vi "room catch or put.vi"(5 "get recy?":bool=TRUE, 7 "first?":bool, 8 "error in (no error)":errorcluster, 9 "Position in":T3, 10 "ff":i32, 11 "main-national data":T1) -> (0 "error out":errorcluster, 1 "Position out":T3, 3 "main-national data out":T1, 4 "finish?":bool)   [LabVIEW 2019]
uses:
  ctl/main data-national.ctl
  ctl/position set.ctl
  subVI/move/position cluster.ctl
  ctl/path name.ctl
  ctl/align type.ctl
  ctl/height.ctl
  ctl/servo act.ctl
panel:
  out "Array":bool[](array[boolean])
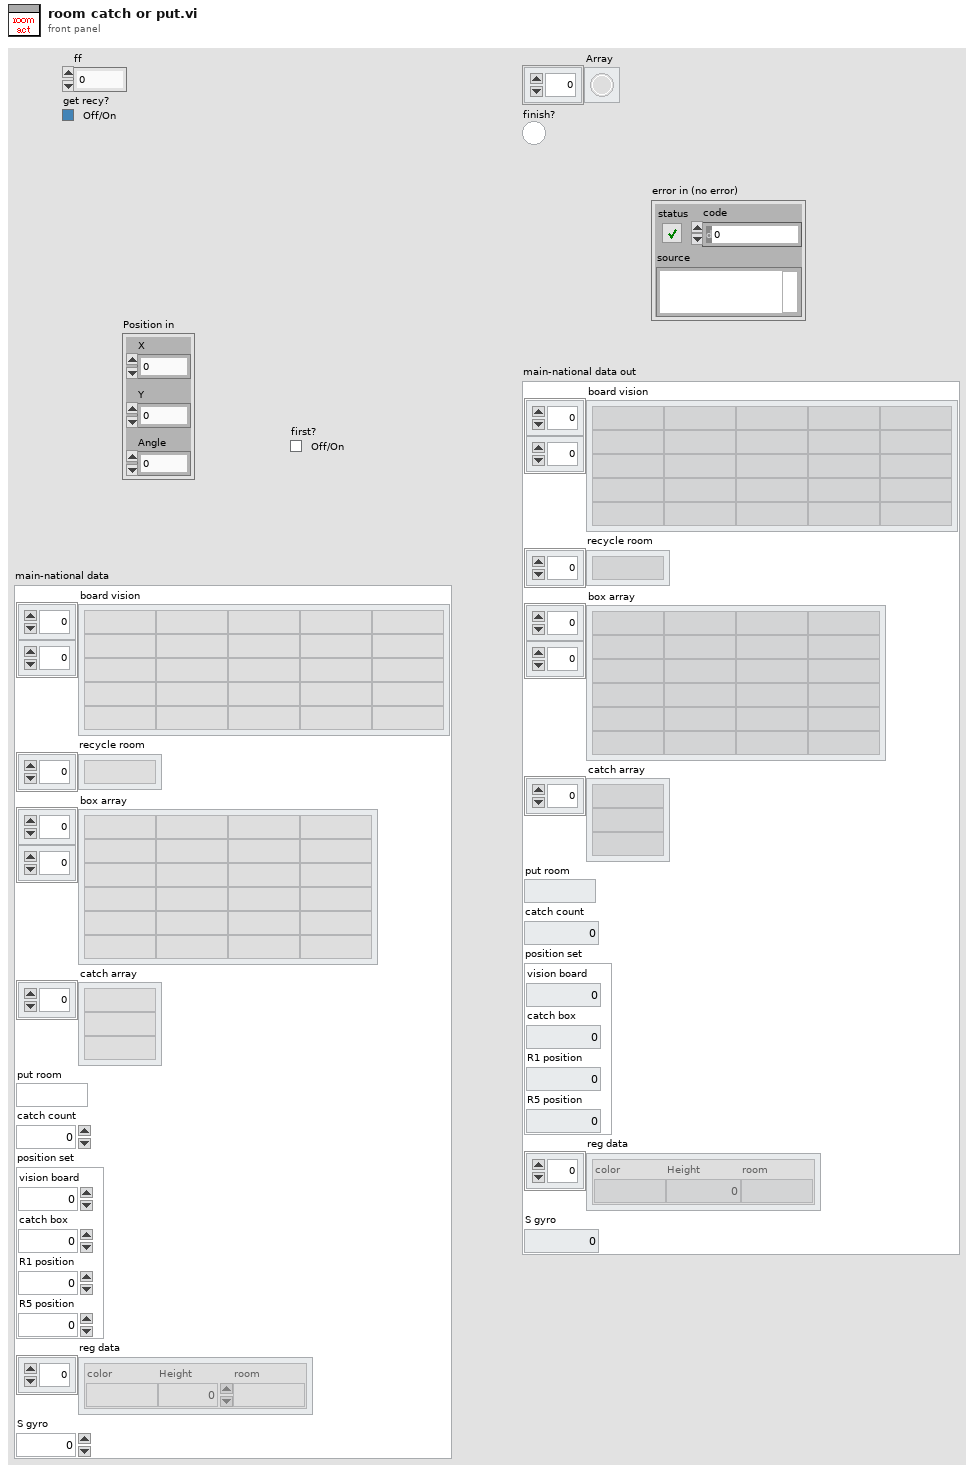
[diagram p1: front panel]
types:
  T1 = typedef "main data-national.ctl" = cluster{"board vision":string[][], "recycle room":string[], "box array":string[][], "catch array":string[], "put room":string, "catch count":dbl, "position set":T2, "reg data":cluster{"color":string, "Height":i32, "room":string}[], "S gyro":dbl}
  T2 = typedef "position set.ctl" = cluster{"vision board":dbl, "catch box":dbl, "R1 position":dbl, "R5 position":dbl}
  T3 = typedef "position cluster.ctl" = cluster{"X":dbl, "Y":dbl, "Angle":dbl}
  T4 = cluster{"color":string, "Height":i32, "room":string}[]
  T5 = typedef "path name.ctl" = enum16{"S - vision board", "vision board - s out", "s out - room center", "room center - R1", "room center - R2", "room center - R3", "room center - R4", "room center - R5", "R1 - room center", "R2 - room center", "R3 - room center", "R4 - room center", "R5 - room center", "room center - S out", "S-out - recycle", "recycle - S-out", "S-out - s", "s - s-out", "board - box", "box - board", "S out - board", "R1 - R1 d", "R5d - R5", "R3.4-R3", "R3 - R3.2", "- align", "- align.5", "R2 - R2.d", "center align"}
  T6 = typedef "align type.ctl" = enum16{"S zone", "box align", "box align contrast", "R1 align", "R5 align", "-> R5 center align", "-> R1 center align"}
  T7 = typedef "servo act.ctl" = enum16{"catch", "relax", "left idle", "center", "red relax", "left reg", "right reg"}
  T8 = typedef "height.ctl" = enum16{"IDLE", "recycle pre-catch", "recycle catch", "recycle zone", "vision height", "box 1", "box 2", "box 3", "box 1 pre", "box 2 pre", "box 3 pre", "reg 1", "reg 2", "reg 1 pre", "reg 2 pre", "put 1", "put 2", "put 3"}
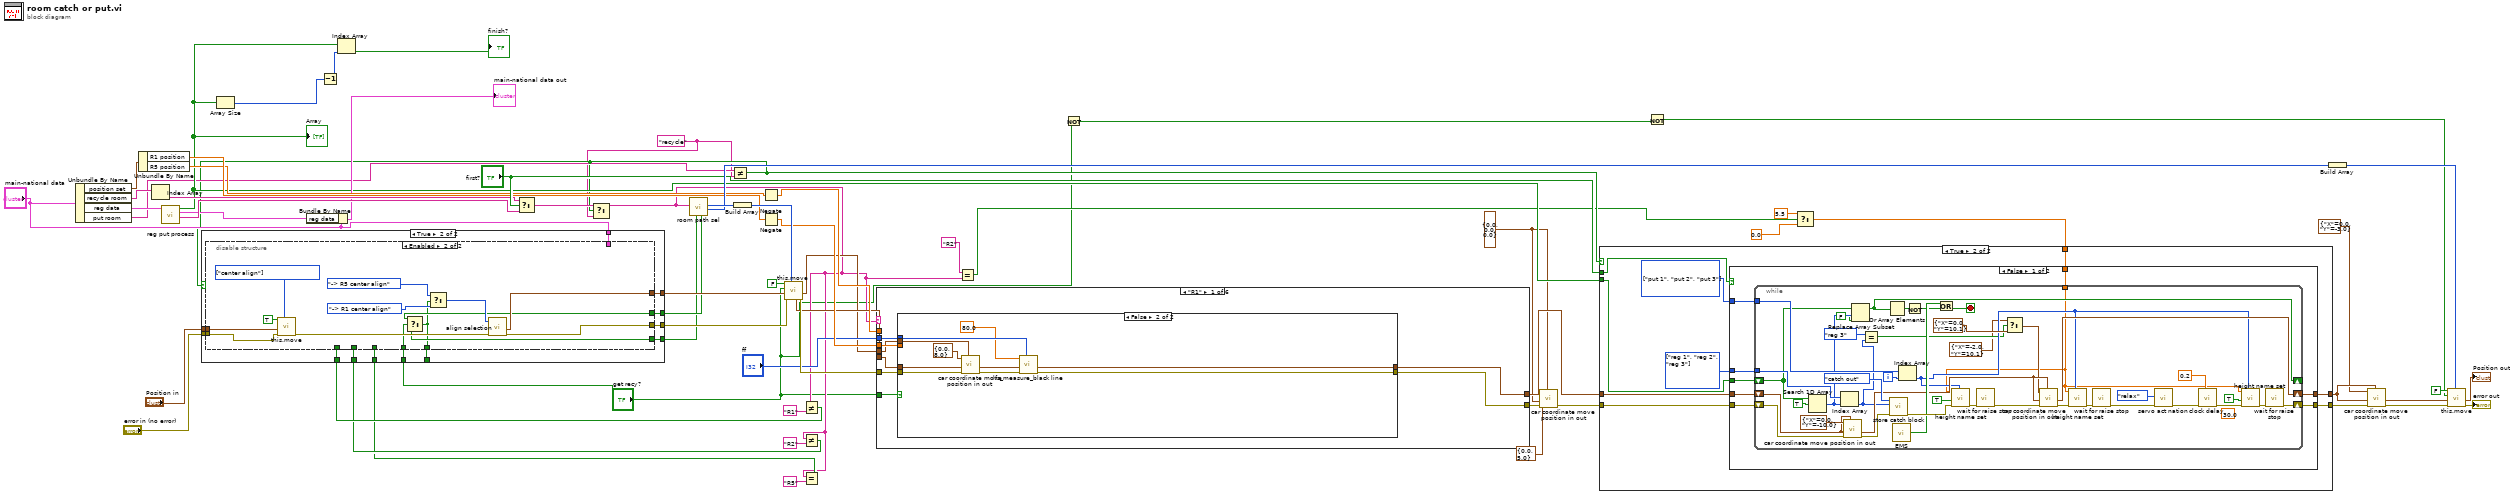
[diagram p0: block diagram]
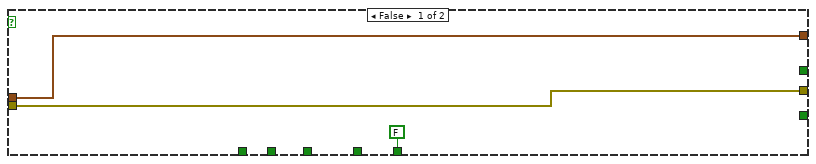
[diagram p2: hidden frame]
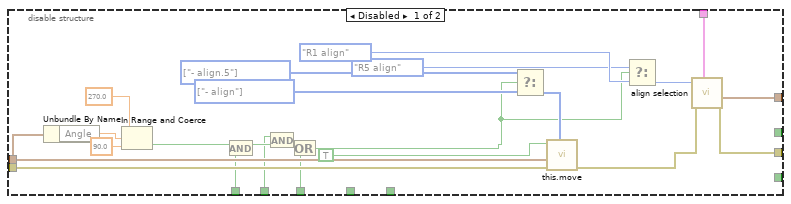
[diagram p3: hidden frame]
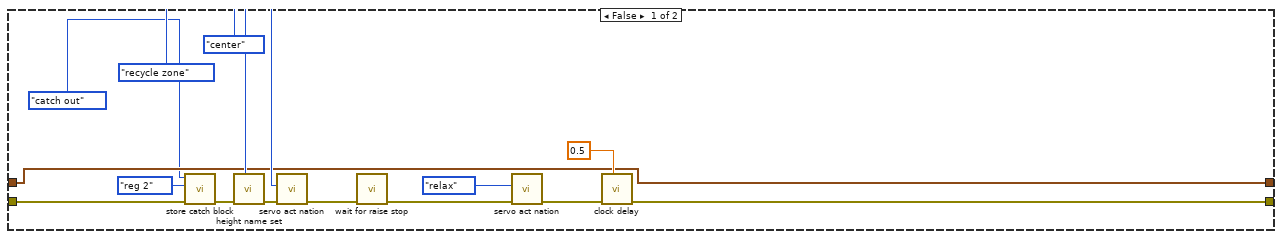
[diagram p4: hidden frame]
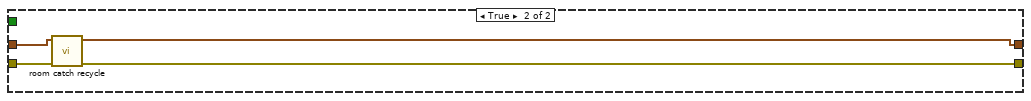
[diagram p5: hidden frame]
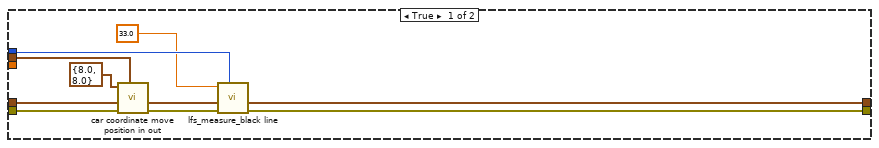
[diagram p6: hidden frame]
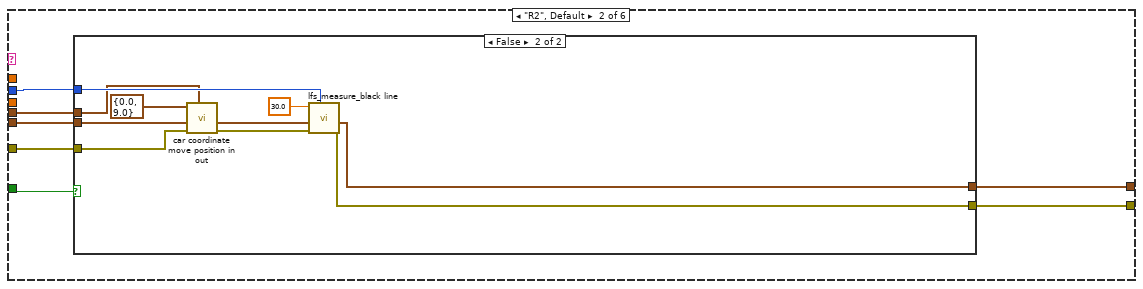
[diagram p7: hidden frame]
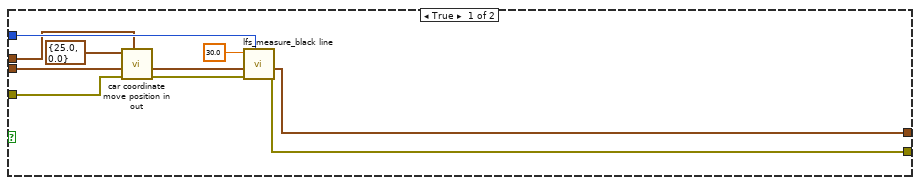
[diagram p8: hidden frame]
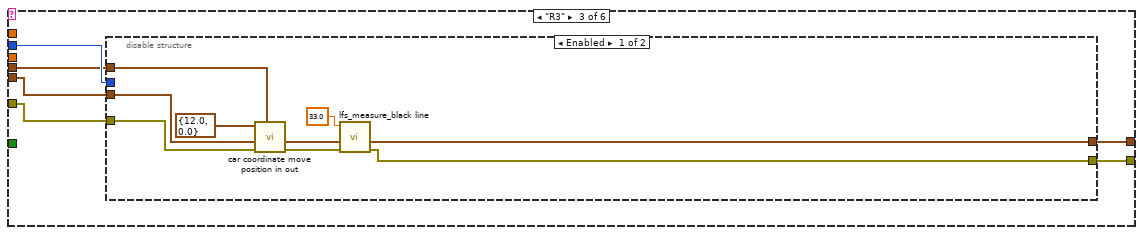
[diagram p9: hidden frame]
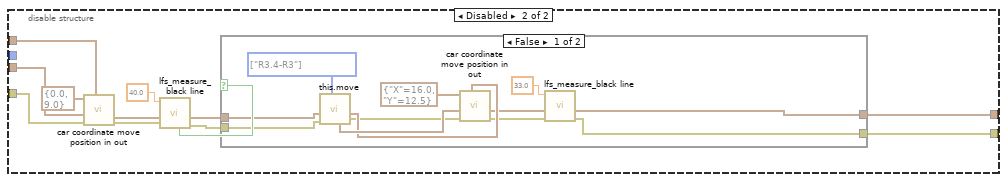
[diagram p10: hidden frame]
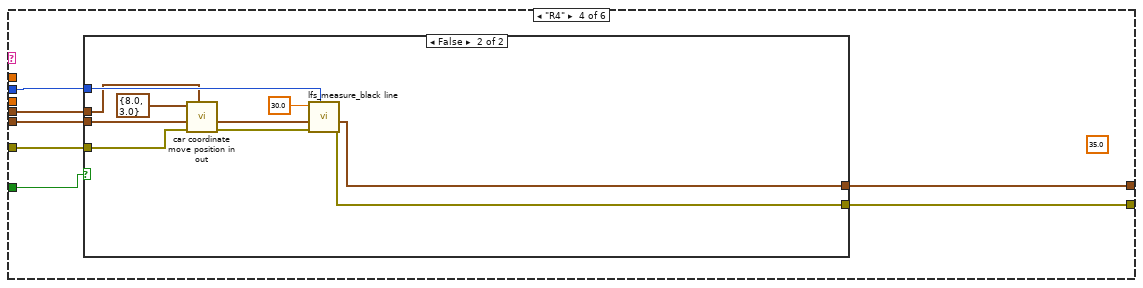
[diagram p12: hidden frame]
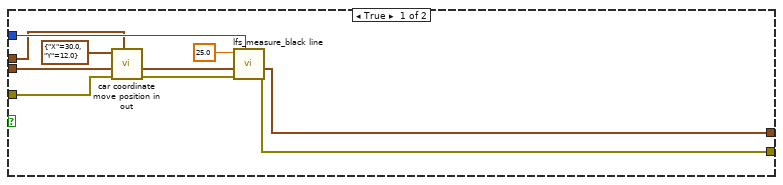
[diagram p13: hidden frame]
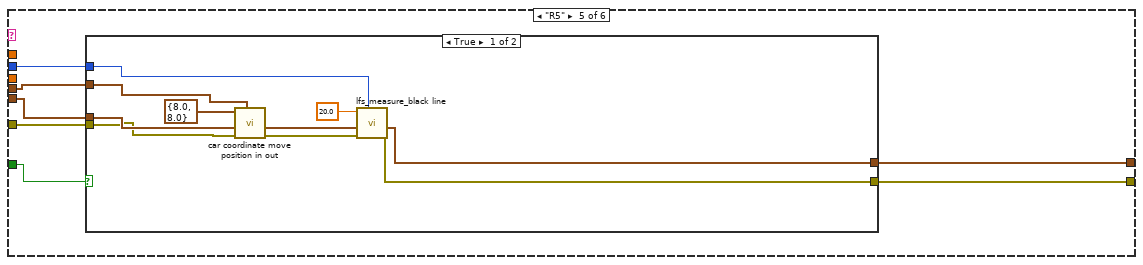
[diagram p14: hidden frame]
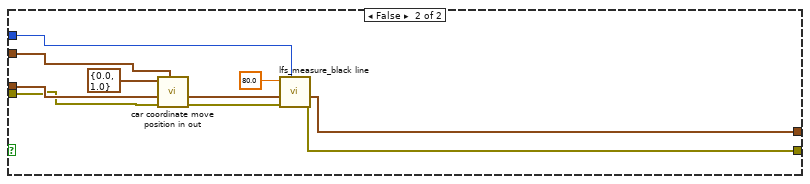
[diagram p15: hidden frame]
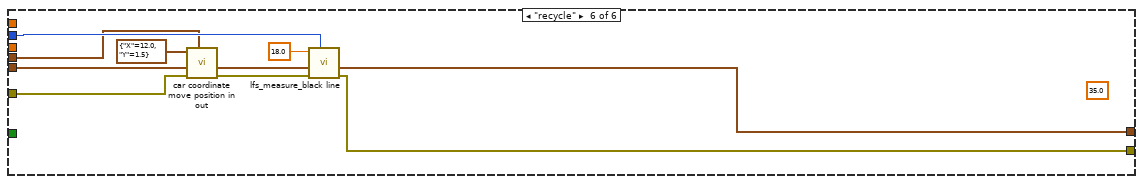
[diagram p16: hidden frame]
diagram:
  w17 = T3 {"X"=0.0, "Y"=0.0, "Angle"=0.0} ("Position in 2")
  w30 = "recycle" ("y")
  n1 = Unbundle By Name("main-national data") -> ("position set"=w52:T2, "recycle room"=w55:string[], "reg data"=w41:T4, "put room"=w32:string)
  n2 = Unbundle By Name(w52) -> ("R1 position"=w51:dbl, "R5 position"=w50:dbl)
  n3 = Index Array(array=w55) -> (element=w47:string)  [unwired: 1 in]
  n4 = call "reg put process.vi"("reg data in"=w41) -> ("room"=w40:string, "reg data out"=w38:T4, "Array"=w34:bool[])  [unwired: 8 in]
  "Array" <- w34
  n5 = Array Size(array=w34) -> (size(s)=w36:i32)
  n6 = Bundle By Name(cluster="main-national data", "reg data"=w38) -> (→"main-national data out":T1)
  n7 = Decrement(x=w36) -> (x-1=w35:i32)
  n8 = Index Array(array=w34, index=w35) -> (element=→"finish?":bool)
  n9 = Select(t=w47, s="first?", f=w40) -> (s? t:f=w53:string)
  n10 = Not Equal?(x=w32, y=w30) -> (x != y?=w31:bool)
  n11 = Select(t=w53, s=w31, f=w30) -> (s? t:f=w10:string)
  n12 = call "room path sel.vi"("room name"=w10) -> ("go next"=w61:T5, "go room path"=w64:T5, "recy dir"=w5:bool, "block dir"=w4:bool)  [unwired: 7 in]
  n13 = Build Array(w64) -> (w63:T5[])
  n14 = Negate(x=w50) -> (-x=w48:dbl)
  n15 = Negate(x=w51) -> (-x=w49:dbl)
  n16 = Not Equal?(x=w10, y="R1") -> (x != y?=w24:bool)
  n17 = Not Equal?(x=w10, y="R2") -> (x != y?=w22:bool)
  n18 = Equal?(x=w10, y="R5") -> (x = y?=w20:bool)
  n19 = case shown="True" w31 {
    tunnel: "Position in" -> [w67 w75]
    tunnel: "error in (no error)" -> [w66 w79]
    tunnel: [w66 w78] -> w43
    tunnel: [w67 w77] -> w42
    tunnel: "main-national data" -> [_ w76]
    tunnel: w24 -> [_ w74]
    tunnel: w22 -> [_ w73]
    tunnel: w20 -> [_ w72]
    tunnel: w5 -> [_ w71]
    tunnel: w4 -> [_ w70]
    tunnel: [FALSE ("block dir") w69] -> _
    tunnel: "get recy?" -> [_ w68]
    frame False {
    }
    frame True {
      n20 = disable-structure shown="Enabled" {
        disable-tunnel: w79 -> [w102 w116]
        disable-tunnel: [w97 w107] -> w78
        disable-tunnel: [w96 w108] -> w77
        disable-tunnel: w76 -> [w95 _]
        disable-tunnel: w75 -> [w92 w115]
        disable-tunnel: w74 -> [w84 _]
        disable-tunnel: w73 -> [w82 _]
        disable-tunnel: w72 -> [w80 _]
        disable-tunnel: w71 -> [_ w106]
        disable-tunnel: w70 -> [_ w105]
        disable-tunnel: [_ w104] -> w69
        disable-tunnel: w68 -> [_ w103]
        frame Disabled {
          w88 = T5[] [enum."- align.5"] items=["S - vision board", "vision board - s out", "s out - room center", "room center - R1", "room center - R2", "room center - R3", "room center - R4", "room center - R5", "R1 - room center", "R2 - room center", "R3 - room center", "R4 - room center", "R5 - room center", "room center - S out", "S-out - recycle", "recycle - S-out", "S-out - s", "s - s-out", "board - box", "box - board", "S out - board", "R1 - R1 d", "R5d - R5", "R3.4-R3", "R3 - R3.2", "- align", "- align.5", "R2 - R2.d", "center align"] ("t")
          w100 = T5[] [enum."- align"] items=["S - vision board", "vision board - s out", "s out - room center", "room center - R1", "room center - R2", "room center - R3", "room center - R4", "room center - R5", "R1 - room center", "R2 - room center", "R3 - room center", "R4 - room center", "R5 - room center", "room center - S out", "S-out - recycle", "recycle - S-out", "S-out - s", "s - s-out", "board - box", "box - board", "S out - board", "R1 - R1 d", "R5d - R5", "R3.4-R3", "R3 - R3.2", "- align", "- align.5", "R2 - R2.d", "center align"] ("path array")
          n21 = Unbundle By Name(w92) -> ("Angle"=w91:dbl)
          n22 = In Range and Coerce(upper limit=270.0, x=w91, lower limit=90.0) -> (In Range?=w87:bool)  [unwired: 1 out]
          n23 = And(x=w87, y=w84) -> (x .and. y?=w85:bool)
          n24 = And(x=w82, y=w85) -> (x .and. y?=w83:bool)
          n25 = Or(x=w83, y=w80) -> (x .or. y?=w81:bool)
          n26 = Select(t=w88, s=w81, f=w100) -> (s? t:f=w93:T5[])
          n27 = call "this.move.vi"("path array"=w93, "error in (no error)"=w102, "Position in"=w92, "enable"=TRUE) -> ("error out"=w98:errorcluster)  [unwired: 4 in, 3 out]
          n28 = Select(t=align_type."R5 align", s=w81, f=align_type."R1 align" ("align type")) -> (s? t:f=w94:T6)
          n29 = call "align selection.vi"("main-national data"=w95, "error in (no error)"=w98, "align type"=w94) -> ("error out"=w97:errorcluster, "Position"=w96:T3)  [unwired: 6 in, 1 out]
        }
        frame Enabled {
          w113 = T5[] [enum."center align"] items=["S - vision board", "vision board - s out", "s out - room center", "room center - R1", "room center - R2", "room center - R3", "room center - R4", "room center - R5", "R1 - room center", "R2 - room center", "R3 - room center", "R4 - room center", "R5 - room center", "room center - S out", "S-out - recycle", "recycle - S-out", "S-out - s", "s - s-out", "board - box", "box - board", "S out - board", "R1 - R1 d", "R5d - R5", "R3.4-R3", "R3 - R3.2", "- align", "- align.5", "R2 - R2.d", "center align"] ("path array")
          n30 = call "this.move.vi"("path array"=w113, "error in (no error)"=w116, "Position in"=w115, "enable"=TRUE) -> ("error out"=w112:errorcluster)  [unwired: 4 in, 3 out]
          n31 = Select(t=w106, s=w103, f=w105) -> (s? t:f=w104:bool)
          n32 = Select(t=align_type."-> R5 center align" ("align type"), s=w104, f=align_type."-> R1 center align" ("align type")) -> (s? t:f=w111:T6)
          n33 = call "align selection.vi"("error in (no error)"=w112, "align type"=w111) -> ("error out"=w107:errorcluster, "Position"=w108:T3)  [unwired: 7 in, 1 out]
        }
      }
    }
  }
  n34 = call "this.move.vi"("path array"=w63, "error in (no error)"=w43, "Position in"=w42, "recy?"="get recy?", "enable"=FALSE) -> ("error out"=w62:errorcluster, "Position out"=w18:T3, "Position out 2"=w19:T3)  [unwired: 3 in, 1 out]
  n35 = case shown="\"R1\"" w10 {
    tunnel: w62 -> [w123 w151 w176 w218 w245 w274]
    tunnel: w19 -> [w124 w150 w177 w219 w246 w275]
    tunnel: [w122 w148 w174 w216 w244 w270] -> w26
    tunnel: [w121 w149 w175 w217 w243 w269] -> w29
    tunnel: w49 -> [w120 _ _ _ _ _]
    tunnel: w48 -> [_ _ _ _ _ _]
    tunnel: "ff" -> [w119 w147 w173 w215 w242 w268]
    tunnel: w18 -> [w118 w146 w172 w214 w241 w267]
    tunnel: "get recy?" -> [w117 w145 _ w213 w240 _]
    frame "R1" {
      n36 = case shown="False" w117 {
        tunnel: w124 -> [w131 w141]
        tunnel: w123 -> [w130 w140]
        tunnel: [w129 w139] -> w122
        tunnel: [w128 w138] -> w121
        tunnel: w120 -> [_ _]
        tunnel: w119 -> [w127 w137]
        tunnel: w118 -> [w126 w136]
        frame True {
          n37 = call "car coordinate move position in out.vi"("Position in 2"=w126, "error in (no error)"=w130, "Position in"=w131, "move"=cluster{"X":dbl, "Y":dbl} {"X"=8.0, "Y"=8.0} ("R1 move")) -> ("error out"=w133:errorcluster, "Position out"=w134:T3)  [unwired: 6 in]
          n38 = call "lfs_measure_black line.vi"("ff"=w127, "error in (no error)"=w133, "Position in"=w134, "limit"=33.0) -> ("error out"=w128:errorcluster, "Position  out"=w129:T3)  [unwired: 3 in, 3 out]
        }
        frame False {
          n39 = call "car coordinate move position in out.vi"("Position in 2"=w136, "error in (no error)"=w140, "Position in"=w141, "move"=cluster{"X":dbl, "Y":dbl} {"X"=0.0, "Y"=8.0} ("R1 move")) -> ("error out"=w143:errorcluster, "Position out"=w144:T3)  [unwired: 6 in]
          n40 = call "lfs_measure_black line.vi"("ff"=w137, "error in (no error)"=w143, "Position in"=w144, "limit"=80.0) -> ("error out"=w138:errorcluster, "Position  out"=w139:T3)  [unwired: 3 in, 3 out]
        }
      }
    }
    frame "R2", Default {
      n41 = case shown="False" w145 {
        tunnel: w151 -> [w161 w171]
        tunnel: w150 -> [w160 w170]
        tunnel: [w159 w169] -> w149
        tunnel: [w158 w168] -> w148
        tunnel: w147 -> [w157 w167]
        tunnel: w146 -> [w156 w166]
        frame True {
          n42 = call "car coordinate move position in out.vi"("Position in 2"=w156, "error in (no error)"=w161, "Position in"=w160, "move"=cluster{"X":dbl, "Y":dbl} {"X"=25.0, "Y"=0.0}) -> ("error out"=w154:errorcluster, "Position out"=w153:T3)  [unwired: 6 in]
          n43 = call "lfs_measure_black line.vi"("ff"=w157, "error in (no error)"=w154, "Position in"=w153, "limit"=30.0) -> ("error out"=w159:errorcluster, "Position  out"=w158:T3)  [unwired: 3 in, 3 out]
        }
        frame False {
          n44 = call "car coordinate move position in out.vi"("Position in 2"=w166, "error in (no error)"=w171, "Position in"=w170, "move"=cluster{"X":dbl, "Y":dbl} {"X"=0.0, "Y"=9.0}) -> ("error out"=w164:errorcluster, "Position out"=w163:T3)  [unwired: 6 in]
          n45 = call "lfs_measure_black line.vi"("ff"=w167, "error in (no error)"=w164, "Position in"=w163, "limit"=30.0) -> ("error out"=w169:errorcluster, "Position  out"=w168:T3)  [unwired: 3 in, 3 out]
        }
      }
    }
    frame "R3" {
      n46 = disable-structure shown="Enabled" {
        disable-tunnel: w177 -> [w182 w197]
        disable-tunnel: w176 -> [w181 w198]
        disable-tunnel: [w180 w188] -> w175
        disable-tunnel: [w179 w187] -> w174
        disable-tunnel: w173 -> [_ _]
        disable-tunnel: w172 -> [w178 w196]
        frame Enabled {
          n47 = call "car coordinate move position in out.vi"("Position in 2"=w178, "error in (no error)"=w181, "Position in"=w182, "move"=cluster{"X":dbl, "Y":dbl} {"X"=12.0, "Y"=0.0}) -> ("error out"=w185:errorcluster, "Position out"=w184:T3)  [unwired: 6 in]
          n48 = call "lfs_measure_black line.vi"("error in (no error)"=w185, "Position in"=w184, "limit"=33.0) -> ("error out"=w180:errorcluster, "Position  out"=w179:T3)  [unwired: 4 in, 3 out]
        }
        frame Disabled {
          n49 = call "car coordinate move position in out.vi"("Position in 2"=w196, "error in (no error)"=w198, "Position in"=w197, "move"=cluster{"X":dbl, "Y":dbl} {"X"=0.0, "Y"=9.0}) -> ("error out"=w192:errorcluster, "Position out"=w193:T3)  [unwired: 6 in]
          n50 = call "lfs_measure_black line.vi"("error in (no error)"=w192, "Position in"=w193, "limit"=40.0) -> ("error out"=w189:errorcluster, "Position  out"=w190:T3, "black?"=w191:bool)  [unwired: 4 in, 2 out]
          n51 = case shown="False" w191 {
            tunnel: w190 -> [w209 w212]
            tunnel: w189 -> [w208 w211]
            tunnel: [w200 w211] -> w188
            tunnel: [w199 w212] -> w187
            frame False {
              w210 = T5[] [enum."R3.4-R3"] items=["S - vision board", "vision board - s out", "s out - room center", "room center - R1", "room center - R2", "room center - R3", "room center - R4", "room center - R5", "R1 - room center", "R2 - room center", "R3 - room center", "R4 - room center", "R5 - room center", "room center - S out", "S-out - recycle", "recycle - S-out", "S-out - s", "s - s-out", "board - box", "box - board", "S out - board", "R1 - R1 d", "R5d - R5", "R3.4-R3", "R3 - R3.2", "- align", "- align.5", "R2 - R2.d", "center align"] ("path array")
              n52 = call "this.move.vi"("path array"=w210, "error in (no error)"=w208, "Position in"=w209) -> ("error out"=w204:errorcluster, "Position out"=w205:T3, "Position out 2"=w206:T3)  [unwired: 5 in, 1 out]
              n53 = call "car coordinate move position in out.vi"("Position in 2"=w205, "error in (no error)"=w204, "Position in"=w206, "move"=cluster{"X":dbl, "Y":dbl} {"X"=16.0, "Y"=12.5}) -> ("error out"=w203:errorcluster, "Position out"=w202:T3)  [unwired: 6 in]
              n54 = call "lfs_measure_black line.vi"("error in (no error)"=w203, "Position in"=w202, "limit"=33.0) -> ("error out"=w200:errorcluster, "Position  out"=w199:T3)  [unwired: 4 in, 3 out]
            }
            frame True {
            }
          }
        }
      }
    }
    frame "R4" {
      (unwired) 35.0 ("speed")
      n55 = case shown="False" w213 {
        tunnel: w219 -> [w225 w235]
        tunnel: w218 -> [w224 w234]
        tunnel: [w223 w233] -> w217
        tunnel: [w222 w232] -> w216
        tunnel: w215 -> [w221 w231]
        tunnel: w214 -> [w220 w230]
        frame True {
          n56 = call "car coordinate move position in out.vi"("Position in 2"=w220, "error in (no error)"=w224, "Position in"=w225, "move"=cluster{"X":dbl, "Y":dbl} {"X"=30.0, "Y"=12.0}) -> ("error out"=w228:errorcluster, "Position out"=w229:T3)  [unwired: 6 in]
          n57 = call "lfs_measure_black line.vi"("ff"=w221, "error in (no error)"=w228, "Position in"=w229, "limit"=25.0) -> ("error out"=w223:errorcluster, "Position  out"=w222:T3)  [unwired: 3 in, 3 out]
        }
        frame False {
          n58 = call "car coordinate move position in out.vi"("Position in 2"=w230, "error in (no error)"=w234, "Position in"=w235, "move"=cluster{"X":dbl, "Y":dbl} {"X"=8.0, "Y"=3.0}) -> ("error out"=w238:errorcluster, "Position out"=w239:T3)  [unwired: 6 in]
          n59 = call "lfs_measure_black line.vi"("ff"=w231, "error in (no error)"=w238, "Position in"=w239, "limit"=30.0) -> ("error out"=w233:errorcluster, "Position  out"=w232:T3)  [unwired: 3 in, 3 out]
        }
      }
    }
    frame "R5" {
      n60 = case shown="True" w240 {
        tunnel: w246 -> [w256 w266]
        tunnel: w245 -> [w255 w265]
        tunnel: [w254 w264] -> w244
        tunnel: [w253 w263] -> w243
        tunnel: w242 -> [w252 w262]
        tunnel: w241 -> [w251 w261]
        frame True {
          n61 = call "car coordinate move position in out.vi"("Position in 2"=w251, "error in (no error)"=w255, "Position in"=w256, "move"=cluster{"X":dbl, "Y":dbl} {"X"=8.0, "Y"=8.0} ("R5 move")) -> ("error out"=w249:errorcluster, "Position out"=w250:T3)  [unwired: 6 in]
          n62 = call "lfs_measure_black line.vi"("ff"=w252, "error in (no error)"=w249, "Position in"=w250, "limit"=20.0 ("R5 limit")) -> ("error out"=w253:errorcluster, "Position  out"=w254:T3)  [unwired: 3 in, 3 out]
        }
        frame False {
          n63 = call "car coordinate move position in out.vi"("Position in 2"=w261, "error in (no error)"=w265, "Position in"=w266, "move"=cluster{"X":dbl, "Y":dbl} {"X"=0.0, "Y"=1.0} ("R5 move")) -> ("error out"=w259:errorcluster, "Position out"=w260:T3)  [unwired: 6 in]
          n64 = call "lfs_measure_black line.vi"("ff"=w262, "error in (no error)"=w259, "Position in"=w260, "limit"=80.0 ("R5 limit")) -> ("error out"=w263:errorcluster, "Position  out"=w264:T3)  [unwired: 3 in, 3 out]
        }
      }
    }
    frame "recycle" {
      (unwired) 35.0 ("speed")
      n65 = call "car coordinate move position in out.vi"("Position in 2"=w267, "error in (no error)"=w274, "Position in"=w275, "move"=cluster{"X":dbl, "Y":dbl} {"X"=12.0, "Y"=1.5}) -> ("error out"=w271:errorcluster, "Position out"=w272:T3)  [unwired: 6 in]
      n66 = call "lfs_measure_black line.vi"("ff"=w268, "error in (no error)"=w271, "Position in"=w272, "limit"=18.0) -> ("error out"=w269:errorcluster, "Position  out"=w270:T3)  [unwired: 3 in, 3 out]
    }
  }
  n67 = Equal?(x="R2", y=w10) -> (x = y?=w9:bool)
  n68 = Not(x="get recy?") -> (.not. x?=w1:bool)
  n69 = call "car coordinate move position in out.vi"("Position in 2"=w17, "error in (no error)"=w29, "Position in"=w17, "move"=cluster{"X":dbl, "Y":dbl} {"X"=0.0, "Y"=5.0}) -> ("error out"=w28:errorcluster)  [unwired: 6 in, 1 out]
  n70 = Not(x=w1) -> (.not. x?=w3:bool)
  n71 = Select(t=5.5, s=w9, f=0.0) -> (s? t:f=w6:dbl)
  n72 = case shown="True" w31 {
    tunnel: w28 -> [w278 w299]
    tunnel: w26 -> [w282 w298]
    tunnel: [w277 w297] -> w16
    tunnel: [w282 w296] -> w15
    tunnel: "first?" -> [_ w295]
    tunnel: w34 -> [_ w292]
    tunnel: w6 -> [_ w291]
    frame False {
      n73 = call "store catch block.vi"("error in"=w278, "reg"=enum16{"reg 1", "reg 2", "reg 3"}."reg 2", "store/catch"=enum16{"store", "catch out"}."catch out") -> ("error out"=w281:errorcluster)  [unwired: 8 in]
      n74 = call "height name set.vi"("height name"=height."recycle zone", "error in (no error)"=w281) -> ("error out"=w289:errorcluster)  [unwired: 9 in]
      n75 = call "servo act nation.vi"("error in"=w289, "servo act"=servo_act."center") -> ("error out"=w287:errorcluster)  [unwired: 9 in]
      n76 = call "wait for raise stop.vi"("Error In"=w287) -> ("Error Out"=w286:errorcluster)  [unwired: 10 in]
      n77 = call "servo act nation.vi"("error in"=w286, "servo act"=servo_act."relax") -> ("error out"=w284:errorcluster)  [unwired: 9 in]
      n78 = call "clock delay.vi"("Delay Time (s)"=0.5, "error in (no error)"=w284) -> ("error out"=w277:errorcluster)  [unwired: 9 in]
    }
    frame True {
      w293 = T8[] [enum."put 1", enum."put 2", enum."put 3"] items=["IDLE", "recycle pre-catch", "recycle catch", "recycle zone", "vision height", "box 1", "box 2", "box 3", "box 1 pre", "box 2 pre", "box 3 pre", "reg 1", "reg 2", "reg 1 pre", "reg 2 pre", "put 1", "put 2", "put 3"] ("height name")
      w294 = enum16{"reg 1", "reg 2", "reg 3"}[] [enum."reg 1", enum."reg 2", enum."reg 3"] items=["reg 1", "reg 2", "reg 3"] ("reg")
      n79 = case shown="False" w295 {
        tunnel: w299 -> [w306 w352]
        tunnel: w298 -> [w307 w351]
        tunnel: [w302 w350] -> w297
        tunnel: [w303 w349] -> w296
        tunnel: w294 -> [w305 _]
        tunnel: w293 -> [w304 _]
        tunnel: w292 -> [w301 _]
        tunnel: w291 -> [w300 _]
        frame False {
          n80 = while {
            shift-right: [w332] -> w303
            shift-left: w307 -> [w317]
            shift-right: [w330] -> w302
            shift-left: w306 -> [w347]
            tunnel: w305 -> [w329]
            tunnel: w304 -> [w336]
            shift-right: [w322] -> _
            shift-left: w301 -> [w325]
            tunnel: w300 -> [w308]
            i -> [w328]
            stop <- w320 stop-if-true
            (unwired) 30.0 ("speed")
            n81 = Search 1D Array(1D array=w325, element=TRUE) -> (index of element=w324:i32)  [unwired: 1 in]
            n82 = Index Array(array=w329, index=w324) -> (element=w312:enum16{"reg 1", "reg 2", "reg 3"})
            n83 = call "car coordinate move position in out.vi"("Position in 2"=w317, "error in (no error)"=w347, "Position in"=w317, "move"=cluster{"X":dbl, "Y":dbl} {"X"=0.0, "Y"=-10.0}) -> ("error out"=w345:errorcluster, "Position out"=w316:T3)  [unwired: 6 in]
            n84 = Replace Array Subset(array=w325, new element=FALSE ("new element/subarray"), index=w324) -> (w322:bool[])
            n85 = Equal?(x=enum16{"reg 1", "reg 2", "reg 3"}."reg 3", y=w312) -> (x = y?=w310:bool)
            n86 = Or Array Elements(Boolean array=w322) -> (logical OR=w321:bool)
            n87 = call "store catch block.vi"("error in"=w345, "reg"=w312, "store/catch"=enum16{"store", "catch out"}."catch out") -> ("error out"=w344:errorcluster)  [unwired: 8 in]
            n88 = call "EMS.vi"() -> ("A/DIO4 (Pin 19)"=w319:bool)
            n89 = Index Array(array=w336, index=w328) -> (element=w313:T8)
            n90 = Not(x=w321) -> (.not. x?=w318:bool)
            n91 = Or(x=w319, y=w318) -> (x .or. y?=w320:bool)
            n92 = call "height name set.vi"("height name"=w313, "error in (no error)"=w344, "plus 2"=TRUE, "offset"=w308) -> ("error out"=w341:errorcluster)  [unwired: 7 in]
            n93 = call "wait for raise stop.vi"("Error In"=w341) -> ("Error Out"=w340:errorcluster)  [unwired: 10 in]
            n94 = Select(t=cluster{"X":dbl, "Y":dbl} {"X"=-2.0, "Y"=10.1} ("move"), s=w310, f=cluster{"X":dbl, "Y":dbl} {"X"=0.0, "Y"=10.1} ("move")) -> (s? t:f=w315:cluster{"X":dbl, "Y":dbl})
            n95 = call "car coordinate move position in out.vi"("Position in 2"=w316, "error in (no error)"=w340, "Position in"=w316, "move"=w315) -> ("error out"=w335:errorcluster, "Position out"=w332:T3)  [unwired: 6 in]
            n96 = call "height name set.vi"("height name"=w313, "error in (no error)"=w335, "offset"=w308) -> ("error out"=w334:errorcluster)  [unwired: 8 in]
            n97 = call "wait for raise stop.vi"("Error In"=w334) -> ("Error Out"=w333:errorcluster)  [unwired: 10 in]
            n98 = call "servo act nation.vi"("error in"=w333, "servo act"=servo_act."relax") -> ("error out"=w339:errorcluster)  [unwired: 9 in]
            n99 = call "clock delay.vi"("Delay Time (s)"=0.2, "error in (no error)"=w339) -> ("error out"=w337:errorcluster)  [unwired: 9 in]
            n100 = call "height name set.vi"("height name"=w313, "error in (no error)"=w337, "plus 2"=TRUE, "offset"=w308) -> ("error out"=w331:errorcluster)  [unwired: 7 in]
            n101 = call "wait for raise stop.vi"("Error In"=w331) -> ("Error Out"=w330:errorcluster)  [unwired: 10 in]
          }
        }
        frame True {
          n102 = call "room catch recycle.vi"("error in (no error)"=w352, "Position in"=w351) -> ("error out"=w350:errorcluster, "Position out"=w349:T3)  [unwired: 8 in]
        }
      }
    }
  }
  n103 = Build Array(w61) -> (w60:T5[])
  n104 = call "car coordinate move position in out.vi"("Position in 2"=w15, "error in (no error)"=w16, "Position in"=w15, "move"=cluster{"X":dbl, "Y":dbl} {"X"=0.0, "Y"=-3.0}) -> ("error out"=w12:errorcluster, "Position out"=w13:T3)  [unwired: 6 in]
  n105 = call "this.move.vi"("path array"=w60, "error in (no error)"=w12, "Position in"=w13, "recy?"=w3, "enable"=FALSE) -> ("error out"=→"error out":errorcluster, "Position out"=→"Position out":T3)  [unwired: 3 in, 2 out]
